vi "Display graph.vi"(0 "Data ip":T1, 5 "Graph reference":T3, 7 "Range (hours)":dbl=2.0, 9 "Range (hours) 2":dbl=48.0, 11 "Range graph3 (hours) in":dbl=2.0 caption="Range (hours)", 12 "Boolean":bool=TRUE caption="Median filter", 13 "Auto-scale \nhorizontal range":bool) -> (4 "Data op":T1, 6 "XY graph":T2)   [LabVIEW 2013]
uses:
  <vilib>/Analysis/NI_AALBase.lvlib
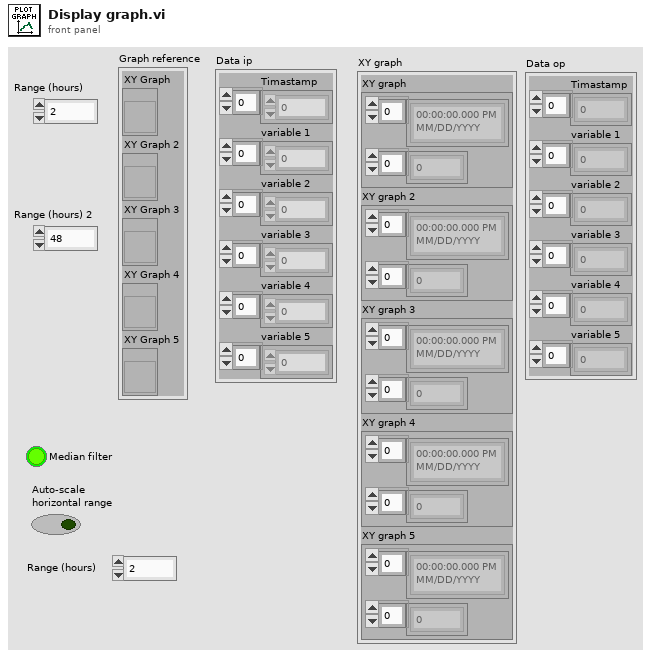
[diagram p1: front panel]
types:
  T1 = cluster{"Timastamp":dbl[], "variable 1":dbl[], "variable 2":dbl[], "variable 3":dbl[], "variable 4":dbl[], "variable 5":dbl[]}
  T2 = cluster{"XY graph":cluster{timestamp[], dbl[]}, "XY graph 2":cluster{timestamp[], dbl[]}, "XY graph 3":cluster{timestamp[], dbl[]}, "XY graph 4":cluster{timestamp[], dbl[]}, "XY graph 5":cluster{timestamp[], dbl[]}}
  T3 = cluster{"XY Graph":refnum<vi>, "XY Graph 2":refnum<vi>, "XY Graph 3":refnum<vi>, "XY Graph 4":refnum<vi>, "XY Graph 5":refnum<vi>}
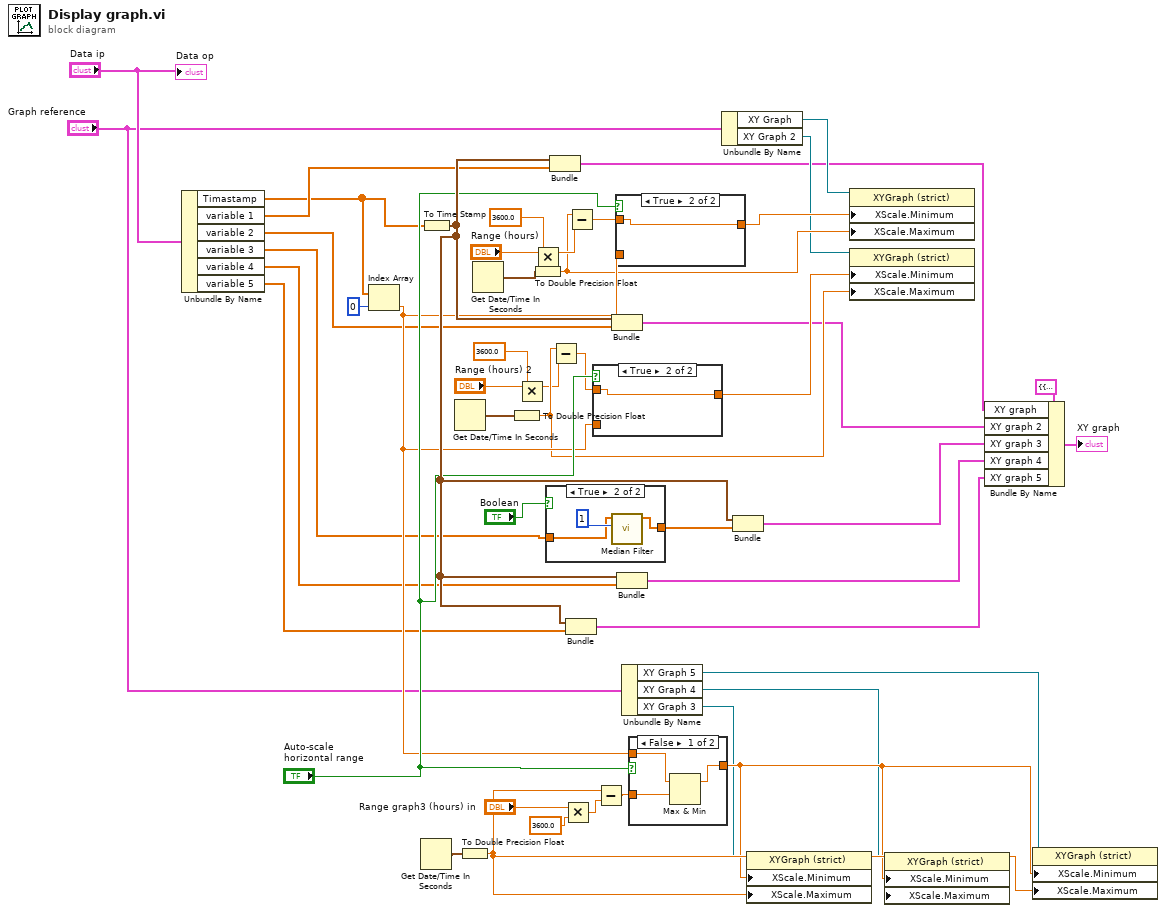
[diagram p0: block diagram]
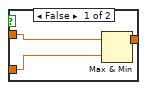
[diagram p3: hidden frame]
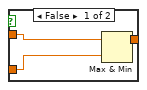
[diagram p4: hidden frame]
diagram:
  n1 = Unbundle By Name("Data ip") -> ("Timastamp"=w14:dbl[], "variable 1"=w19:dbl[], "variable 2"=w18:dbl[], "variable 3"=w17:dbl[], "variable 4"=w16:dbl[], "variable 5"=w15:dbl[])
  n2 = Index Array(array=w14, index=0) -> (element=w41:dbl)
  n3 = Get Date/Time In Seconds() -> (seconds since 1Jan1904=w31:timestamp)
  n4 = To Time Stamp(1:w14) -> (0:w43:timestamp[])
  n5 = Get Date/Time In Seconds() -> (seconds since 1Jan1904=w29:timestamp)
  n6 = To Double Precision Float(number=w31) -> (double precision float=w45:dbl)
  n7 = Get Date/Time In Seconds() -> (seconds since 1Jan1904=w21:timestamp)
  n8 = To Double Precision Float(number=w29) -> (double precision float=w30:dbl)
  n9 = Multiply(x="Range (hours) 2", y=3600.0) -> (x*y=w27:dbl)
  n10 = Multiply(x="Range (hours)", y=3600.0) -> (x*y=w24:dbl)
  n11 = To Double Precision Float(number=w21) -> (double precision float=w23:dbl)
  n12 = case shown="True" "Boolean" {
    tunnel: w17 -> [w48 w50]
    tunnel: [w48 w49] -> w46
    frame False {
    }
    frame True {
      n13 = call <vilib>:"Median Filter.vi"("left rank"=1, "X"=w50) -> ("Filtered X"=w49:dbl[])  [unwired: 8 in, 1 out]
    }
  }
  n14 = Bundle(w43, "variable 1"=w19) -> (w7:cluster{timestamp[], "variable 1":dbl[]})  [unwired: 1 in]
  n15 = Subtract(x=w30, y=w27) -> (x-y=w40:dbl)
  n16 = Multiply(x="Range graph3 (hours) in", y=3600.0) -> (x*y=w33:dbl)
  n17 = Bundle(w43, "variable 5"=w15) -> (w3:cluster{timestamp[], "variable 5":dbl[]})  [unwired: 1 in]
  n18 = Subtract(x=w23, y=w24) -> (x-y=w37:dbl)
  n19 = case shown="True" "Auto-scale \nhorizontal range" {
    tunnel: w40 -> [w53 w55]
    tunnel: w41 -> [w52 _]
    tunnel: [w54 w55] -> w39
    frame False {
      n20 = Max & Min(x=w53, y=w52) -> (max(x,y)=w54:dbl)  [unwired: 1 out]
    }
    frame True {
    }
  }
  n21 = Subtract(x=w45, y=w33) -> (x-y=w36:dbl)
  n22 = Bundle(w43, "variable 2"=w18) -> (w6:cluster{timestamp[], "variable 2":dbl[]})  [unwired: 1 in]
  n23 = case shown="True" "Auto-scale \nhorizontal range" {
    tunnel: w37 -> [w57 w59]
    tunnel: w41 -> [w56 _]
    tunnel: [w58 w59] -> w38
    frame False {
      n24 = Max & Min(x=w57, y=w56) -> (max(x,y)=w58:dbl)  [unwired: 1 out]
    }
    frame True {
    }
  }
  n25 = Bundle(w43, "variable 4"=w16) -> (w4:cluster{timestamp[], "variable 4":dbl[]})  [unwired: 1 in]
  n26 = Unbundle By Name("Graph reference") -> ("XY Graph 5"=w9:refnum<vi>, "XY Graph 4"=w10:refnum<vi>, "XY Graph 3"=w11:refnum<vi>)
  n27 = case shown="False" "Auto-scale \nhorizontal range" {
    tunnel: w41 -> [w61 _]
    tunnel: w36 -> [w60 w63]
    tunnel: [w62 w63] -> w44
    frame False {
      n28 = Max & Min(x=w61, y=w60) -> (max(x,y)=w62:dbl)  [unwired: 1 out]
    }
    frame True {
    }
  }
  n29 = Unbundle By Name("Graph reference") -> ("XY Graph"=w13:refnum<vi>, "XY Graph 2"=w12:refnum<vi>)
  n30 = Bundle(w43, "Filtered X"=w46) -> (w5:cluster{timestamp[], "Filtered X":dbl[]})  [unwired: 1 in]
  n31 = property on="Property Node" class="XYGraph (strict)"(reference=w11, "XScale.Minimum"=w44, "XScale.Maximum"=w45) -> ()  [unwired: 1 in, 2 out]
  n32 = property on="Property Node" class="XYGraph (strict)"(reference=w13, "XScale.Minimum"=w38, "XScale.Maximum"=w23) -> ()  [unwired: 1 in, 2 out]
  n33 = property on="Property Node" class="XYGraph (strict)"(reference=w12, "XScale.Minimum"=w39, "XScale.Maximum"=w30) -> ()  [unwired: 1 in, 2 out]
  n34 = property on="Property Node" class="XYGraph (strict)"(reference=w10, "XScale.Minimum"=w44, "XScale.Maximum"=w45) -> ()  [unwired: 1 in, 2 out]
  n35 = Bundle By Name(cluster=T2 {"XY graph"={[], []}, "XY graph 2"={[], []}, "XY graph 3"={[], []}, "XY graph 4"={[], []}, "XY graph 5"={[], []}}, "XY graph"=w7, "XY graph 2"=w6, "XY graph 3"=w5, "XY graph 4"=w4, "XY graph 5"=w3) -> (→"XY graph":T2)
  n36 = property on="Property Node" class="XYGraph (strict)"(reference=w9, "XScale.Minimum"=w44, "XScale.Maximum"=w45) -> ()  [unwired: 1 in, 2 out]
  "Data op" <- "Data ip"
